vi "SubVI - Send Report Files.vi"(8 "error in":errorcluster, 11 "File Path":path) -> (0 "error out":errorcluster)   [LabVIEW 2017]
panel:
  out "x-y":dbl
  out "Timer":u32
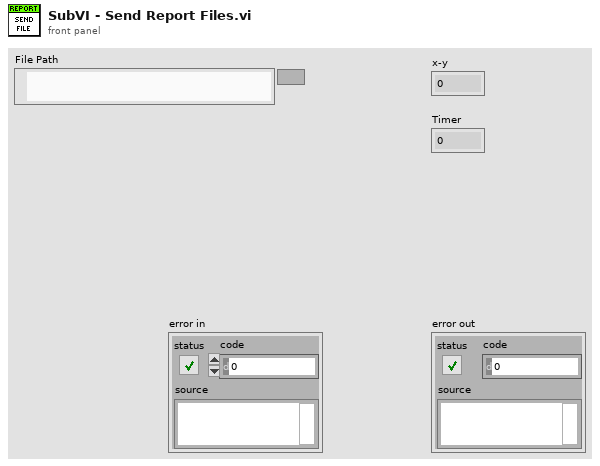
[diagram p1: front panel]
types:
  T1 = enum16{"big-endian, network order", "native, host order", "little-endian"}
  T2 = enum16{"open", "replace", "create", "open or create", "replace or create", "replace or create with confirmation"}
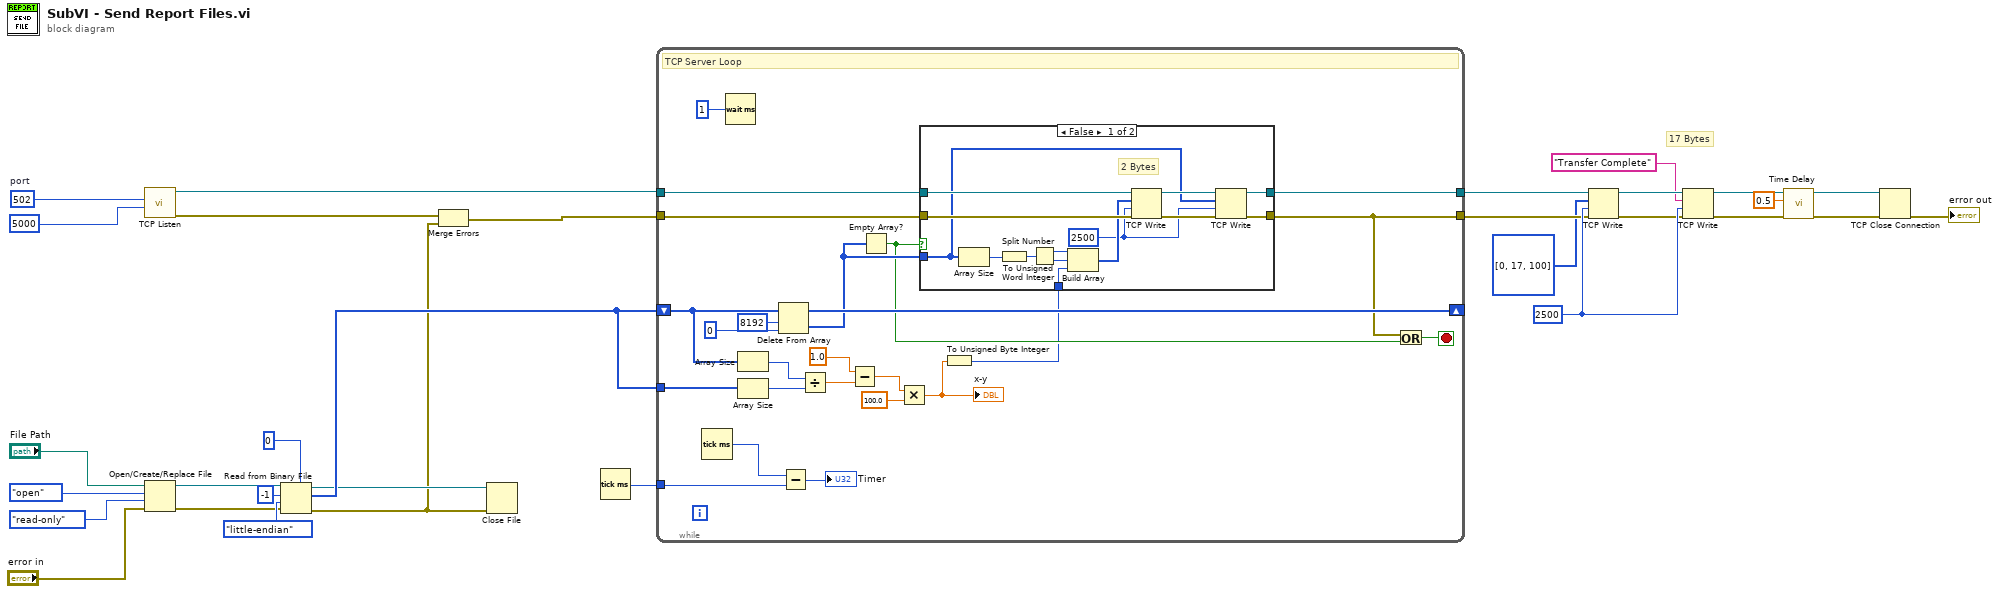
[diagram p0: block diagram]
diagram:
  w30 = 2500 ("timeout ms (25000)")
  w16 = u16 502  # port
  # "17 Bytes"
  n1 = call <vilib>:"TCP Listen.vi"("timeout ms (wait forever: -1)"=5000, "port"=w16) -> ("error out"=w3:errorcluster, "connection ID"=w22:refnum<k5>)  [unwired: 5 in, 3 out]
  n2 = Open/Create/Replace File(file path (use dialog)="File Path", error in="error in", operation (0:open)=T2."open", access (0:read/write)=enum16{"read/write", "read-only", "write-only"}."read-only") -> (refnum out=w8:refnum<file>, error out=w9:errorcluster)  [unwired: 2 in, 1 out]
  n3 = Read from Binary File(5:u8 0, 8:w9, 9:T1."little-endian" ("byte order (0:big-endian, network order)"), 10:-1 ("count (1)"), 11:w8) -> (0:w2:errorcluster, 2:w28:u8[], 3:w10:refnum<file>)  [unwired: 1 in, 1 out]
  n4 = Merge Errors(w3, w2) -> (w1:errorcluster)
  n5 = Close File(refnum=w10, error in=w2) -> ()  [unwired: 2 out]
  n6 = Tick Count (ms)() -> (millisecond timer value=w29:u32)
  n7 = while {
    tunnel: w1 -> [w46]
    tunnel: w22 -> [w47]
    tunnel: [w53] -> w24
    tunnel: [w48] -> w25
    shift-right: [w50] -> _
    shift-left: w28 -> [w42]
    tunnel: w28 -> [w43]
    tunnel: w29 -> [w34]
    stop <- w49 stop-if-true
    # "TCP Server Loop"
    n8 = Tick Count (ms)() -> (millisecond timer value=w35:u32)
    n9 = Wait (ms)(milliseconds to wait=u32 1) -> ()  [unwired: 1 out]
    n10 = Array Size(array=w42) -> (size(s)=w40:i32)
    n11 = Array Size(array=w43) -> (size(s)=w41:i32)
    n12 = Delete From Array(array=w42, length=8192, index=0) -> (deleted portion=w45:u8[], array with subset deleted=w50:u8[])
    n13 = Subtract(x=w35, y=w34) -> (x-y=→"Timer":u32)
    n14 = Divide(x=w40, y=w41) -> (x/y=w38:dbl)
    n15 = Subtract(x=1.0, y=w38) -> (x-y=w37:dbl)
    n16 = Empty Array?(array=w45) -> (empty?=w44:bool)
    n17 = Multiply(x=w37, y=100.0) -> (x*y=w32:dbl)
    "x-y" <- w32
    n18 = To Unsigned Byte Integer(number=w32) -> (unsigned 8bit integer=w31:u8)
    n19 = case shown="False" w44 {
      tunnel: [w68 w70] -> w53
      tunnel: [w67 w69] -> w48
      tunnel: w47 -> [w66 w70]
      tunnel: w46 -> [w64 w69]
      tunnel: w45 -> [w62 _]
      tunnel: w31 -> [w55 _]
      frame False {
        w56 = 2500 ("timeout ms (25000)")
        # "2 Bytes"
        n20 = Array Size(array=w62) -> (size(s)=w61:i32)
        n21 = To Unsigned Word Integer(number=w61) -> (unsigned 16bit integer=w60:u16)
        n22 = Split Number(x=w60) -> (hi(x)=w59:u8, lo(x)=w58:u8)
        n23 = Build Array(w59, w58, w55) -> (w57:u8[])
        n24 = TCP Write(connection ID=w66, data in=w57, error in (no error)=w64, 9:w56) -> (connection ID out=w65:refnum<k5>, error out=w63:errorcluster)  [unwired: 1 out]
        n25 = TCP Write(connection ID=w65, data in=w62, error in (no error)=w63, 9:w56) -> (connection ID out=w68:refnum<k5>, error out=w67:errorcluster)  [unwired: 1 out]
      }
      frame True {
      }
    }
    n26 = Or(x=w48, y=w44) -> (x .or. y?=w49:bool)
  }
  n27 = TCP Write(connection ID=w24, data in=u8[] [0, 17, 100], error in (no error)=w25, 9:w30) -> (connection ID out=w26:refnum<k5>, error out=w27:errorcluster)  [unwired: 1 out]
  n28 = TCP Write(connection ID=w26, data in="Transfer Complete", error in (no error)=w27, 9:w30) -> (connection ID out=w15:refnum<k5>, error out=w20:errorcluster)  [unwired: 1 out]
  n29 = call "Time Delay"("error in (no error)"=w20, "Delay Time (s)"=0.5) -> ("error out"=w21:errorcluster)  [unwired: 9 in]
  n30 = TCP Close Connection(connection ID=w15, error in (no error)=w21) -> (error out=→"error out":errorcluster)  [unwired: 1 in, 1 out]
